vi "Get Object by Type.vi"(7 "Object Type":refnum<class>, 8 "error in (no error)":errorcluster, 11 "Processing in":refnum<class "Processing.lvclass">) -> (0 "error out":errorcluster, 2 "Object":refnum<class>, 3 "Processing out":refnum<class "Processing.lvclass">)   [LabVIEW 2020, in "HTTP Server.lvlib" / "Processing.lvclass"]
uses:
  Processing.lvclass
  Processing.lvclass/Processing.ctl
  Values/Values.lvclass
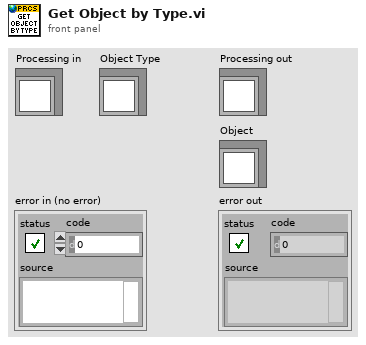
[diagram p1: front panel]
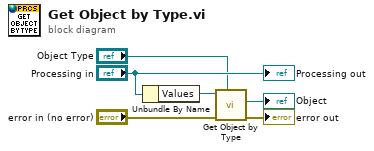
[diagram p0: block diagram]
diagram:
  n1 = Unbundle By Name("Processing in") -> ("Values"=w5:refnum<class "Values.lvclass">)
  n2 = call "Get Object by Type.vi"("Object Type"="Object Type", "error in (no error)"="error in (no error)", "Values in"=w5) -> ("error out"=→"error out":errorcluster, "Object"=→"Object":refnum<class>)  [unwired: 6 in, 1 out]
  "Processing out" <- "Processing in"
